vi "Configure Make Digitize Measurement.vi"(6 "Buffer Name (\"defbuffer1\")":string="defbuffer1", 8 "error in (no error)":errorcluster, 9 "Readings Count (1)":u32=1, 10 "Block Number (0)":u32, 11 "VISA resource name":refnum<visa-resource-name>) -> (0 "error out":errorcluster, 3 "VISA resource name out":refnum<visa-resource-name>)   [LabVIEW 2016, in "Keithley DMM6500 DAQ6500 Series.lvlib"]
doc: "Branches to a specified block when a specified trigger event occurs."
uses:
  Keithley DMM6500 DAQ6500 Series.lvlib
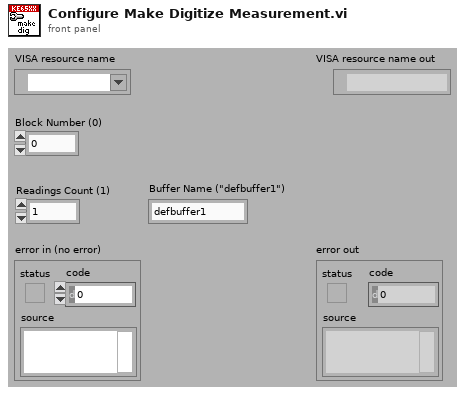
[diagram p1: front panel]
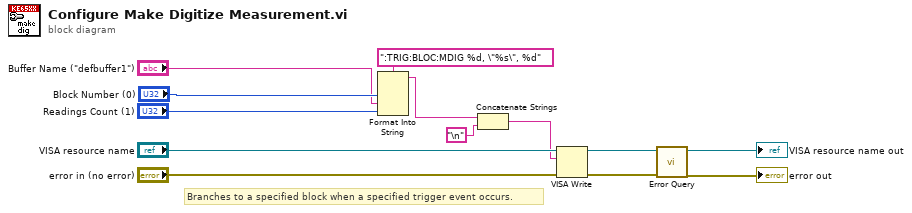
[diagram p0: block diagram]
diagram:
  # "Branches to a specified block when a specified trigger event occurs."
  n1 = Format Into String(format string=":TRIG:BLOC:MDIG %d, \"%s\", %d", "Block Number (0)", "Buffer Name (\"defbuffer1\")", "Readings Count (1)") -> (resulting string=w2:string)  [unwired: 2 in, 1 out]
  n2 = Concatenate Strings(w2, "\n") -> (w3:string)
  n3 = VISA Write(VISA resource name="VISA resource name", write buffer=w3, error in (no error)="error in (no error)") -> (VISA resource name out=w7:refnum<visa-resource-name>, error out=w6:errorcluster)  [unwired: 1 out]
  n4 = call "Error Query.vi"("error in (no error)"=w6, "VISA resource name"=w7) -> ("error out"=→"error out":errorcluster, "VISA resource name out"=→"VISA resource name out":refnum<visa-resource-name>)  [unwired: 6 in, 2 out]
